vi "Insert_2Event_Log(Trigger).vi"(8 "data":string="790", 9 "message":string="B", 10 "output cluster":cluster{"barcode A":string, "barcode B":string}, 11 "DBlink":string="Driver={ODBC Driver 17 for SQL Server};Server=localhost\\SQLEXPRESS;Database=ZDX201;UID=labview;PWD=Dsa@54137926") -> ()   [LabVIEW 2019]
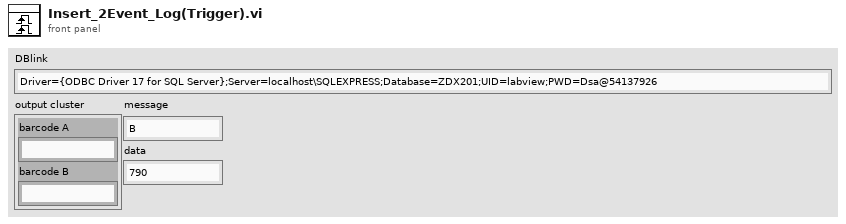
[diagram p1: front panel]
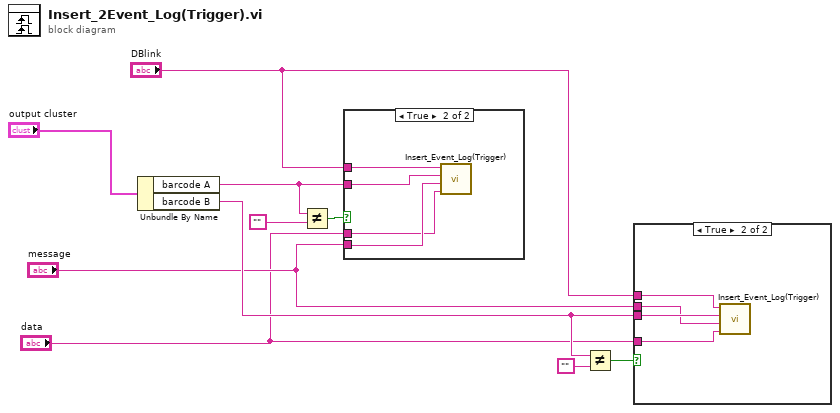
[diagram p0: block diagram]
diagram:
  n1 = Unbundle By Name("output cluster") -> ("barcode A"=w6:string, "barcode B"=w5:string)
  n2 = Not Equal?(x=w6, y="") -> (x != y?=w7:bool)
  n3 = case shown="True" w7 {
    tunnel: "DBlink" -> [_ w14]
    tunnel: w6 -> [_ w12]
    tunnel: "message" -> [_ w13]
    tunnel: "data" -> [_ w11]
    frame False {
    }
    frame True {
      n4 = call "Insert_Event_Log(Trigger).vi"("data"=w11, "message"=w13, "id"=w12, "DBlink"=w14) -> ()  [unwired: 8 in]
    }
  }
  n5 = Not Equal?(x=w5, y="") -> (x != y?=w3:bool)
  n6 = case shown="True" w3 {
    tunnel: w5 -> [_ w18]
    tunnel: "DBlink" -> [_ w17]
    tunnel: "message" -> [_ w16]
    tunnel: "data" -> [_ w15]
    frame False {
    }
    frame True {
      n7 = call "Insert_Event_Log(Trigger).vi"("data"=w15, "message"=w16, "id"=w18, "DBlink"=w17) -> ()  [unwired: 8 in]
    }
  }
